vi "sub_get_list_of_waveforms.vi"(8 "error in":errorcluster, 11 "daq.io type in":T1={"daq.io ref"=refnum, "daq.io API Base"="", "Device Type Key"="", "Device Key"="", "Account ID"="", "online"=FALSE, "SSL"=TRUE}) -> (0 "error out":errorcluster, 1 "Waveform base URI":string, 2 "Existing Waveforms":T3[](array[typedef]), 3 "daq.io type out":T1={"daq.io ref"=refnum, "daq.io API Base"="", "Device Type Key"="", "Device Key"="", "Account ID"="", "online"=FALSE, "SSL"=TRUE})   [LabVIEW 2013, in "daqio minimal.lvlib"]
doc: "This VI retrieves all Waveform entries for a specified device. It will not download the actual data but rather the header information. With the \"ID\" that this VI returns, the actual waveform data can be retrieved."
uses:
  daqio minimal.lvlib
  _typedefs/daqio-read-waveform-JSON-header-time.ctl
  _typedefs/daqio-Type.ctl
  <vilib>/httpClient/ClientHandle.ctl
  _typedefs/daqio-read-waveform-JSON-header.ctl
  _typedefs/FGV_commands.ctl
  <vilib>/Easy HTTP Client/Easy HTTP.lvlib
  <vilib>/httpClient/LabVIEWHTTPClient.lvlib
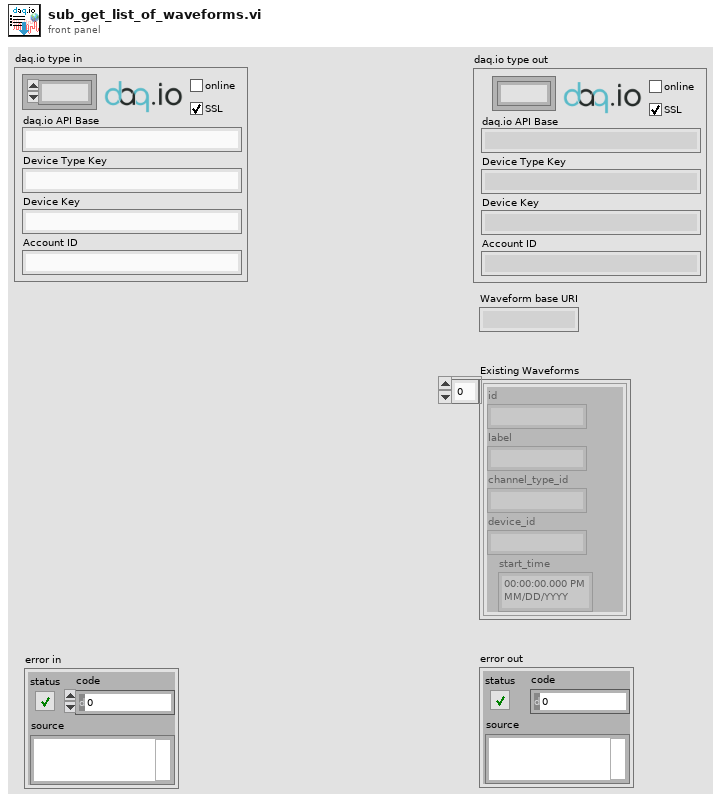
[diagram p1: front panel]
types:
  T1 = typedef "daqio minimal.lvlib/daqio-Type.ctl" = cluster{"daq.io ref":T2, "daq.io API Base":string, "Device Type Key":string, "Device Key":string, "Account ID":string, "online":bool, "SSL":bool}
  T2 = typedef "LabVIEWHTTPClient.lvlib/ClientHandle.ctl" = refnum<k1>
  T3 = typedef "daqio minimal.lvlib/daqio-read-waveform-JSON-header-time.ctl" = cluster{"id":string, "label":string, "channel_type_id":string, "device_id":string, "start_time":timestamp}
  T4 = typedef "daqio minimal.lvlib/FGV_commands.ctl" = enum16{"Init / Update", "Read From File", "Edit Item", "Find or Add Item", "Remove Item", "Delete All"}
  T5 = typedef "daqio minimal.lvlib/daqio-read-waveform-JSON-header.ctl" = cluster{"id":string, "label":string, "channel_type_id":string, "device_id":string, "start_time":string}
  T6 = typedef "daqio minimal.lvlib/daqio-Device-Type-Info-return.ctl" = cluster{"channel_types":T7[], "devices":T8[], "label":string, "event_types":T9[], "key":string, "tag_types":T10[], "id":string, "permissions":cluster{"write":string[], "read":string[]}}
  T7 = typedef "daqio minimal.lvlib/daqio-Channel-Type-POST-return.ctl" = cluster{"device_type_id":string, "id":string, "key":string, "label":string, "data_type":string, "permissions":cluster{"write":string[], "read":string[]}}
  T8 = typedef "daqio minimal.lvlib/daqio-Device.ctl" = cluster{"permissions":cluster{"write":string[], "read":string[]}, "id":string, "label":string, "key":string, "device_type_id":string, "tags":cluster{"key":string, "value":string}[], "files":string[]}
  T9 = typedef "daqio minimal.lvlib/daqio-Event-Type.ctl" = cluster{"device_type_id":string, "permissions":cluster{"read":string[], "write":string[]}, "id":string, "key":string, "label":string}
  T10 = typedef "daqio minimal.lvlib/daqio-Tag-Type-POST-return.ctl" = cluster{"label":string, "id":string, "device_type_id":string, "permissions":cluster{"write":string[], "read":string[]}, "default":string, "key":string}
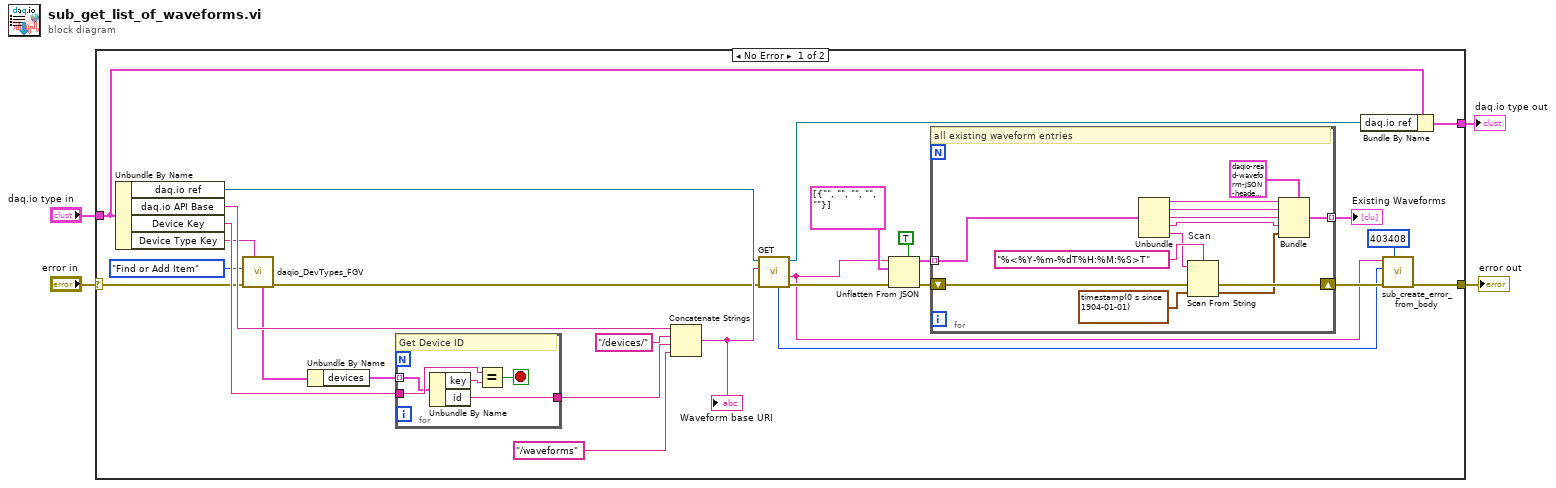
[diagram p0: block diagram]
diagram:
  n1 = case shown="No Error" "error in" {
    selector: "error in" -> [w13 w50]
    tunnel: "daq.io type in" -> [w12 w51]
    tunnel: [w10 w51] -> w2
    tunnel: [w6 w50] -> w1
    frame No Error {
      n2 = Unbundle By Name(w12) -> ("daq.io ref"=w14:T2, "daq.io API Base"=w25:string, "Device Key"=w24:string, "Device Type Key"=w21:string)
      n3 = call "daqio_DevTypes_FGV.vi"("Dev Type Key"=w21, "error in (no error)"=w13, "Action"=FGV_commands."Find or Add Item") -> ("error out"=w27:errorcluster, "Dev Type out"=w22:T6)  [unwired: 4 in, 3 out]
      n4 = Unbundle By Name(w22) -> ("devices"=w23:T8[])
      n5 = for {
        tunnel: w23 -> [w34] mode=indexing
        tunnel: w24 -> [w36]
        tunnel: [w32] -> w28
        stop <- w35 stop-if-true
        # "Get Device ID"
        n6 = Unbundle By Name(w34) -> ("key"=w33:string, "id"=w32:string)
        n7 = Equal?(x=w36, y=w33) -> (x = y?=w35:bool)
      }
      n8 = Concatenate Strings(w25, "/devices/" ("string"), w28, "/waveforms" ("string")) -> (w30:string)
      "Waveform base URI" <- w30
      n9 = call <vilib>:"GET.vi"("error in (no error)"=w27, "url"=w30, "client handle"=w14) -> ("error out"=w15:errorcluster, "body"=w7:string, "client handle out"=w11:T2, "HTTP Response Code"=w8:i32)  [unwired: 4 in, 1 out]
      n10 = Unflatten From JSON(enable LabVIEW extensions? (T)=TRUE, JSON string=w7, type and defaults=T5[] [{"id"="", "label"="", "channel_type_id"="", "device_id"="", "start_time"=""}], error in (no error)=w15) -> (value=w17:T5[], error out=w18:errorcluster)  [unwired: 3 in]
      n11 = for {
        tunnel: w17 -> [w45] mode=indexing
        shift-right: [w46] -> w9
        shift-left: w18 -> [w47]
        tunnel: [w37] -> w31 mode=indexing
        # "all existing waveform entries"
        n12 = Unbundle(w45) -> ("id"=w42:string, "label"=w41:string, "channel_type_id"=w40:string, "device_id"=w39:string, "start_time"=w44:string)
        n13 = Scan From String "Scan"(format string="%<%Y-%m-%dT%H:%M:%S>T" ("input string"), input string=w44, error in=w47, default 1=timestamp(0 s since 1904-01-01) ("default value 1")) -> (error out=w46:errorcluster, output 1=w38:timestamp)  [unwired: 1 in, 2 out]
        n14 = Bundle(cluster=T3 {"id"="", "label"="", "channel_type_id"="", "device_id"="", "start_time"=timestamp(0 s since 1904-01-01)} ("Waveform"), "id"=w42, "label"=w41, "channel_type_id"=w40, "device_id"=w39, "start_time"=w38) -> (w37:T3)
      }
      "Existing Waveforms" <- w31
      n15 = Bundle By Name(cluster=w12, "daq.io ref"=w11) -> (w10:T1)
      n16 = call "sub_create_error_from_body.vi"("error code"=403408, "error in (no error)"=w9, "http code"=w8, "body"=w7) -> ("error out"=w6:errorcluster)  [unwired: 7 in]
    }
    frame Error {
    }
  }
  "daq.io type out" <- w2
  "error out" <- w1
